vi "z_stack_waveform.vi"(4 "Z stack backward":cluster{"采样率":dbl, "采样数":dbl}={"采样率"=50000.0, "采样数"=7000.0}, 6 "Z stack acquisition":cluster{"采样率":dbl, "采样数":dbl}={"采样率"=50000.0, "采样数"=13000.0}, 7 "Steps per Volume":dbl=25.0, 9 "Backward Time (s)":dbl=0.14, 10 "SPECIFIC scan volt":dbl=5.0, 11 "Aquisition Time (s)":dbl=0.26) -> (3 "WaveformOut":waveform(dbl))   [LabVIEW 2018]
uses:
  <vilib>/Waveform/WDTOps.llb/WDT Append Waveforms DBL.vi
  <vilib>/measure/NI_MABase.lvlib
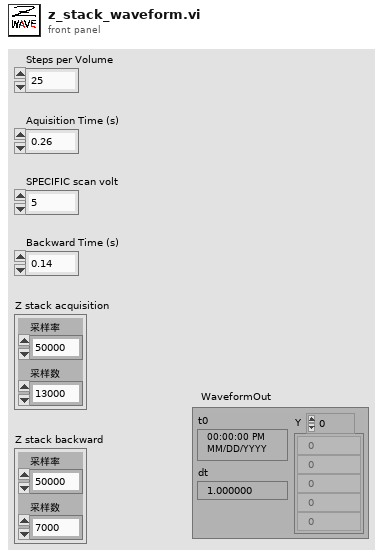
[diagram p1: front panel]
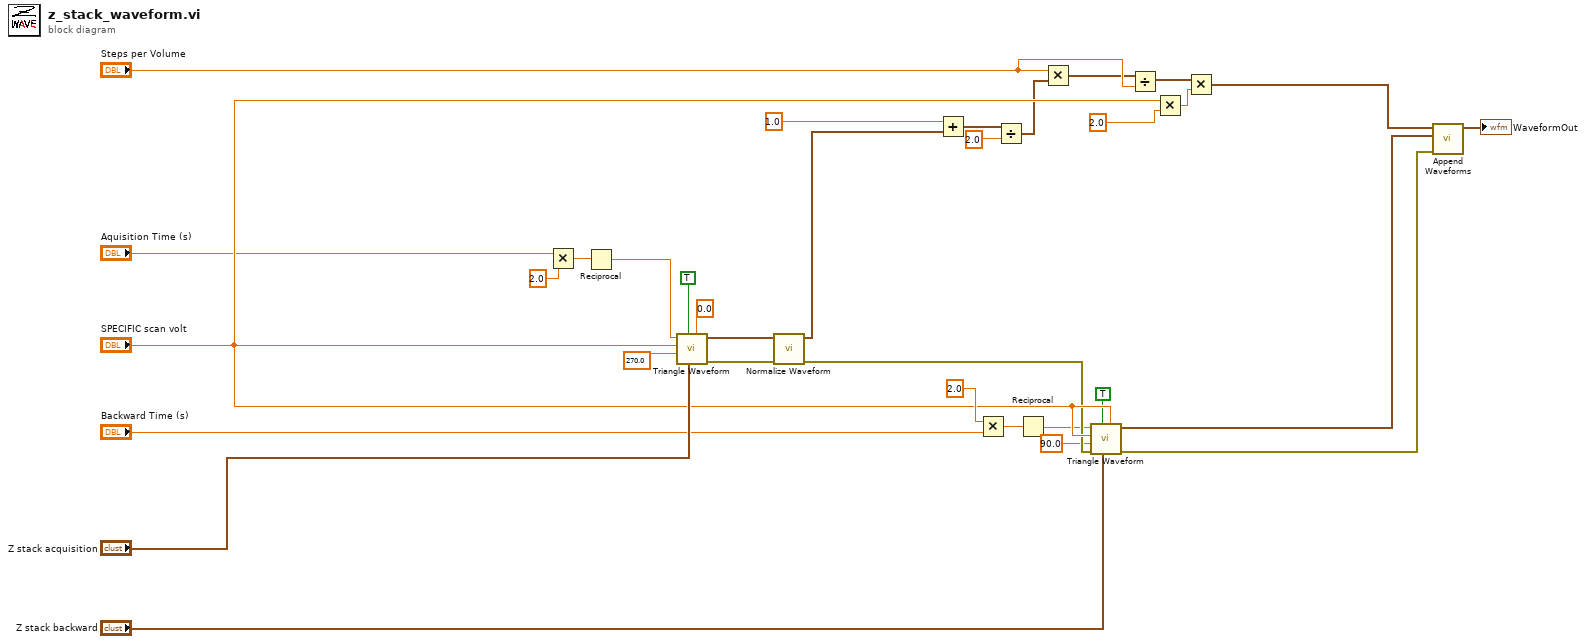
[diagram p0: block diagram]
diagram:
  n1 = Multiply(x="Aquisition Time (s)", y=2.0) -> (x*y=w7:dbl)
  n2 = Reciprocal(x=w7) -> (1/x=w8:dbl)
  n3 = call <vilib>:"Triangle Waveform.vi"("offset"=0.0, "sampling info"="Z stack acquisition", "reset signal"=TRUE, "phase"=270.0, "amplitude"="SPECIFIC scan volt", "frequency"=w8) -> ("error out"=w12:errorcluster, "signal out"=w4:waveform(dbl))  [unwired: 4 in]
  n4 = call <vilib>:"Normalize Waveform.vi"("error in (no error)"=w12, "waveform in"=w4) -> ("error out"=w27:errorcluster, "normalized waveform"=w13:waveform(dbl))  [unwired: 6 in, 2 out]
  n5 = Add(x=1.0 ("offset"), y=w13) -> (x+y=w15:waveform(dbl))
  n6 = Multiply(x=2.0 ("y"), y="Backward Time (s)") -> (x*y=w24:dbl)
  n7 = Divide(x=w15, y=2.0 ("offset")) -> (x/y=w17:waveform(dbl))
  n8 = Reciprocal(x=w24) -> (1/x=w25:dbl)
  n9 = Multiply(x="Steps per Volume", y=w17) -> (x*y=w18:waveform(dbl))
  n10 = call <vilib>:"Triangle Waveform.vi"("offset"="SPECIFIC scan volt", "sampling info"="Z stack backward", "reset signal"=TRUE, "error in (no error)"=w27, "phase"=90.0, "amplitude"="SPECIFIC scan volt", "frequency"=w25) -> ("error out"=w28:errorcluster, "signal out"=w2:waveform(dbl))  [unwired: 3 in]
  n11 = Divide(x=w18, y="Steps per Volume") -> (x/y=w20:waveform(dbl))
  n12 = Multiply(x="SPECIFIC scan volt", y=2.0) -> (x*y=w21:dbl)
  n13 = Multiply(x=w20, y=w21) -> (x*y=w3:waveform(dbl))
  n14 = call-poly <vilib>:"Append Waveforms.vi"("error in (no error)"=w28, "waveform B"=w2, "waveform A"=w3) -> ("waveform out"=→"WaveformOut":waveform(dbl))  [unwired: 7 in, 1 out]
